vi "Message-handler.vi"(8 "error in (no error)":errorcluster, 11 "Client in":T1) -> (0 "error out":errorcluster, 3 "Client out":T1)   [LabVIEW 2013, in "Client.lvlib" / "Client.lvclass"]
doc: "Simple example of a continuous communication monitor loop.\nThe function continuously monitors the incomming (client) communication channel. At regular intervals, or after receiving a message, the client activity is reaffirmed through a 'heartbeat' message to the server.\nA new message is handled through the 'Process-received-message' function, which checks the message origins, determines the appropriate client action and executes this action."
uses:
  Client.lvclass
  Object-reference.ctl
  Supported-actions.ctl
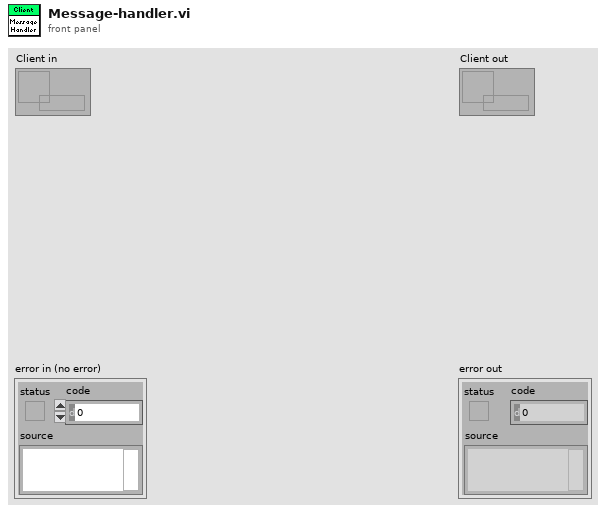
[diagram p1: front panel]
types:
  T1 = typedef "Client.lvlib/Client.lvclass/Object-reference.ctl" = refnum<data-value>
  T2 = typedef "Client.lvlib/Client.lvclass/Supported-actions.ctl" = enum16{"Idle", "Initialize", "Load settings", "Load file", "Ready", "Start", "Pause", "Stop", "Repeat", "Reset", "Exit"}
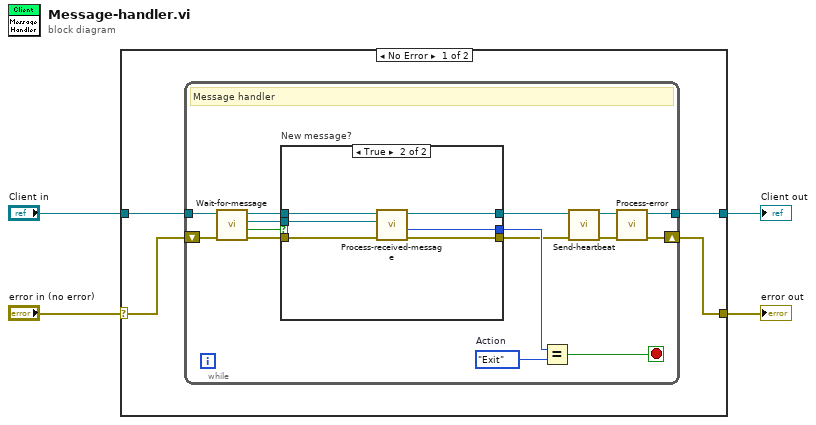
[diagram p0: block diagram]
diagram:
  n1 = case shown="No Error" "error in (no error)" {
    selector: "error in (no error)" -> [w6 w33]
    tunnel: [w5 w33] -> w3
    tunnel: [w7 w32] -> w1
    tunnel: "Client in" -> [w8 w32]
    frame No Error {
      n2 = while {
        tunnel: w8 -> [w23]
        tunnel: [w16] -> w7
        shift-right: [w17] -> w5
        shift-left: w6 -> [w21]
        stop <- w15 stop-if-true
        w14 = Supported-actions."Exit"  # Action
        # "Message handler"
        n3 = call "Wait-for-message.vi"("error in (no error)"=w21, "Client in"=w23) -> ("error out"=w20:errorcluster, "New message?"=w18:bool, "Message"=w19:refnum<class "Message.lvclass">, "Client out"=w22:T1)  [unwired: 6 in]
        n4 = case "New message?" shown="True" w18 {
          tunnel: w22 -> [w25 w31]
          tunnel: [w25 w30] -> w12
          tunnel: w20 -> [w24 w29]
          tunnel: w19 -> [_ w28]
          tunnel: [w24 w27] -> w10
          tunnel: [_ w26] -> w13
          frame False {
          }
          frame True {
            n5 = call "Process-received-message.vi"("error in (no error)"=w29, "Message"=w28, "Client in"=w31) -> ("error out"=w27:errorcluster, "Action"=w26:T2, "Client out"=w30:T1)  [unwired: 6 in]
          }
        }
        n6 = Equal?(x=w13, y=w14) -> (x = y?=w15:bool)
        n7 = call "Send-heartbeat.vi"("error in (no error)"=w10, "Client in"=w12) -> ("error out"=w9:errorcluster, "Client out"=w11:T1)  [unwired: 8 in]
        n8 = call "Process-error.vi"("error in (no error)"=w9, "Client in"=w11) -> ("error out"=w17:errorcluster, "Client out"=w16:T1)  [unwired: 8 in]
      }
    }
    frame Error {
    }
  }
  "error out" <- w3
  "Client out" <- w1
